vi "Start Process.vi"(8 "error in (no error)":errorcluster, 11 "CoolApp in":refnum<class "CoolApp.lvclass">) -> (0 "error out":errorcluster, 3 "CoolApp out":refnum<class "CoolApp.lvclass">)   [LabVIEW 2020, in "LAF2024Q2.lvlib" / "CoolApp.lvclass"]
uses:
  CoolApp.lvclass
  C:/dev/lv 2020/laf-2024-q2/LAF2024Q2/CoolAppProcess/CoolAppProcess.lvclass
  ChartProc/ChartProc.lvclass
  DAQProc/DAQProc.lvclass
  Nested.ctl
  <vilib>/ActorFramework/Message Enqueuer/Message Enqueuer.lvclass
  CoolApp.lvclass/CoolApp.ctl
  CoolAppProcess/CoolAppProcess.lvclass
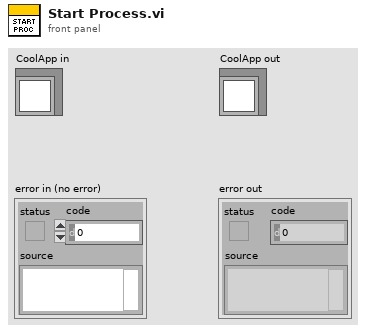
[diagram p1: front panel]
types:
  T1 = typedef "LAF2024Q2.lvlib/CoolApp.lvclass/Nested.ctl" = enum16{"DAQ", "Chart"}
  T2 = map{refnum<class "Message Enqueuer.lvclass">, T1}
  T3 = map{T1, refnum<class "Message Enqueuer.lvclass">}
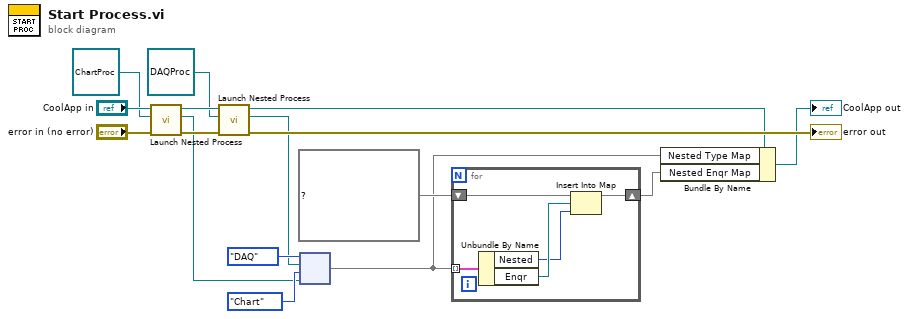
[diagram p0: block diagram]
diagram:
  n1 = call "Launch Nested Process.vi"("error in (no error)"="error in (no error)", "Nested"=refnum<class "ChartProc.lvclass"> refnum ("LAF2024Q2.lvlib:ChartProc.lvclass"), "CoolAppProcess in"="CoolApp in") -> ("error out"=w15:errorcluster, "Enqr"=w5:refnum<class "Message Enqueuer.lvclass">, "CoolAppProcess out"=w11:refnum<class "CoolApp.lvclass">)  [unwired: 6 in]
  n2 = call "Launch Nested Process.vi"("error in (no error)"=w15, "Nested"=refnum<class "DAQProc.lvclass"> refnum ("LAF2024Q2.lvlib:DAQProc.lvclass"), "CoolAppProcess in"=w11) -> ("error out"=→"error out":errorcluster, "Enqr"=w7:refnum<class "Message Enqueuer.lvclass">, "CoolAppProcess out"=w10:refnum<class "CoolApp.lvclass">)  [unwired: 6 in]
  n3 = node(Nested."DAQ" ("Nested"), w7, Nested."Chart" ("Nested"), w5) -> (w1:T3)
  n4 = for {
    tunnel: w1 -> [w21] mode=indexing
    shift-right: [w17] -> w2
    shift-left: T2 {} ("Nested Enqr Map") -> [w18]
    n5 = Unbundle By Name(w21) -> ("Nested"=w19:T1, "Enqr"=w20:refnum<class "Message Enqueuer.lvclass">)
    n6 = Insert Into Map(map in=w18, key=w20, value=w19) -> (map out=w17:T2)  [unwired: 2 out]
  }
  n7 = Bundle By Name(cluster=w10, "Nested Type Map"=w1, "Nested Enqr Map"=w2) -> (→"CoolApp out":refnum<class "CoolApp.lvclass">)
